vi "GlobalVi.vi"() -> ()   [LabVIEW 2015]
panel:
  out "Washer":bool
  out "QAQCvacoff":bool
  out "PinInsertGlue":bool
  out "QAQCvacon":bool
  out "StiffRemoval":bool
  out "DryRunFull":bool
  out "AllCoolBar":bool
  out "AddHoneycomb":bool
  out "AddFrame":bool
  out "DryRunEmpty":bool
  out "PCBalignStiff":bool
  out "PCBposStiff":bool
  out "PCBalignTab":bool
  out "NewPanel":bool
  out "panelTest":bool
  out "countdown":bool
  out "closePanel":bool
  out "stbackPCBglue":bool
  out "innerStructure":bool
  out "tablePCBglue":bool
  out "stbackTest":bool
  out "stbackPCBtest":bool
  out "tablePCBtest":bool
  in  "dimbar":T1={"top"=0, "left"=235, "bottom"=900, "right"=1024}
  in  "dimvertmenu":T1={"top"=0, "left"=0, "bottom"=900, "right"=235}
  in  "dimsmall":T1={"top"=0, "left"=235, "bottom"=650, "right"=1024}
  in  "dimbig":T1={"top"=0, "left"=235, "bottom"=900, "right"=1024}
  out "PCBposTab":bool
  # "Checks not used anymore"
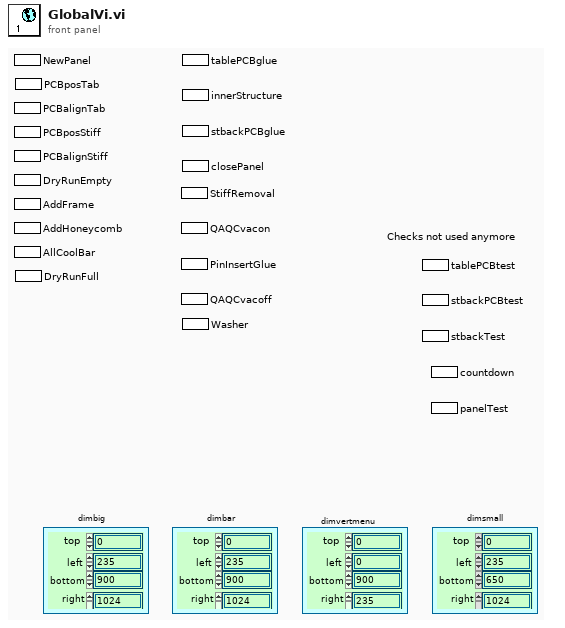
[diagram p1: front panel]
types:
  T1 = cluster{"top":i32, "left":i32, "bottom":i32, "right":i32}
diagram:
